vi "UIDatabaseAdapter.vi"(8 "error in (no error)":errorcluster, 10 "UI Data":variant, 11 "RequestRestUI in":refnum<class "RequestRestUI.lvclass">=refnum) -> (0 "error out":errorcluster, 2 "Database Data":variant, 3 "RequestRestUI out":refnum<class "RequestRestUI.lvclass">)   [LabVIEW 2015, in "UserManagement.lvlib" / "RequestRestMember.lvclass"]
uses:
  UserManagement/Emengency/RequestRestMember.lvclass
  typedef/RequestRestInfo.ctl
  RequestRestUI.lvclass
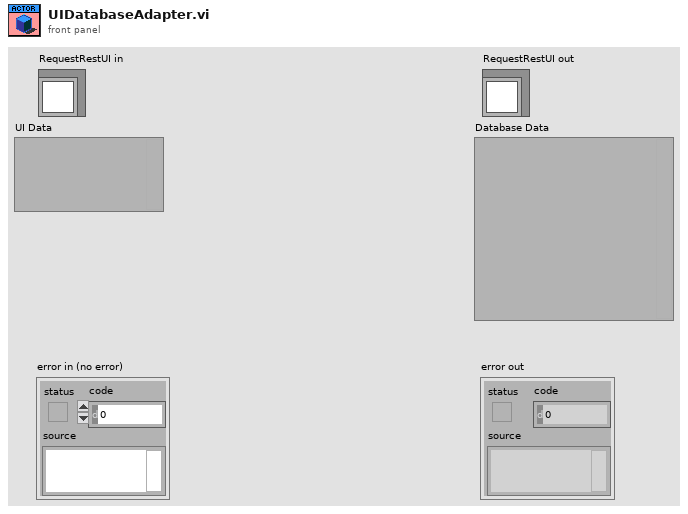
[diagram p1: front panel]
types:
  T1 = typedef "RequestRestUI.lvclass/RequestRestInfo.ctl" = cluster{"学号":string, "姓名":string, "开始时间":timestamp, "结束时间":timestamp, "请假理由":string}
  T2 = cluster{"学号":string, "姓名":string, "date/time string":string, "date/time string":string, "请假理由":string}
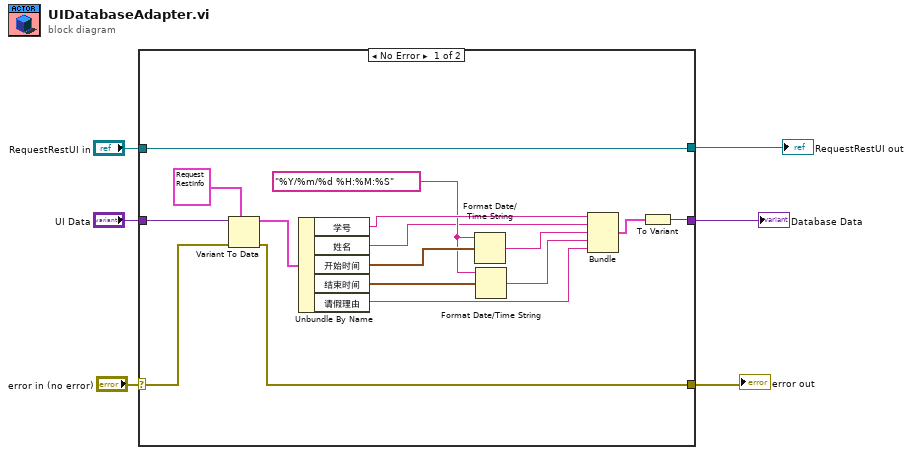
[diagram p0: block diagram]
diagram:
  n1 = case shown="No Error" "error in (no error)" {
    selector: "error in (no error)" -> [w20 w23]
    tunnel: "RequestRestUI in" -> [w22 w25]
    tunnel: "UI Data" -> [w21 w24]
    tunnel: [w22 w25] -> w3
    tunnel: [w10 w24] -> w1
    tunnel: [w9 w23] -> w2
    frame No Error {
      w8 = "%Y/%m/%d %H:%M:%S" ("time format string (%c)")
      n2 = Variant To Data(error in=w20, type=T1 {"学号"="", "姓名"="", "开始时间"=timestamp(0 s since 1904-01-01), "结束时间"=timestamp(0 s since 1904-01-01), "请假理由"=""} ("请假内容"), Variant=w21) -> (data=w18:T1, error out=w9:errorcluster)
      n3 = Unbundle By Name(w18) -> ("学号"=w16:string, "姓名"=w7:string, "开始时间"=w17:timestamp, "结束时间"=w14:timestamp, "请假理由"=w12:string)
      n4 = Format Date/Time String(time format string (%c)=w8, seconds (now)=w17) -> (date/time string=w15:string)  [unwired: 1 in]
      n5 = Format Date/Time String(time format string (%c)=w8, seconds (now)=w14) -> (date/time string=w13:string)  [unwired: 1 in]
      n6 = Bundle("学号"=w16, "姓名"=w7, "date/time string"=w15, "date/time string"=w13, "请假理由"=w12) -> (w11:T2)  [unwired: 1 in]
      n7 = To Variant(anything=w11) -> (Variant=w10:variant)
    }
    frame Error {
    }
  }
  "error out" <- w2
  "RequestRestUI out" <- w3
  "Database Data" <- w1
